vi "Save Data.vi"(0 "Which Button?":T1(ring)=enum."Center Button", 1 "start path":path, 5 "Header (If NEW is selected)":string, 7 "Data to be saved (String)":string, 9 "default name":string, 11 "error in (no error)":errorcluster) -> (4 "Maybe go back?":bool, 15 "error out":errorcluster)   [LabVIEW 2020]
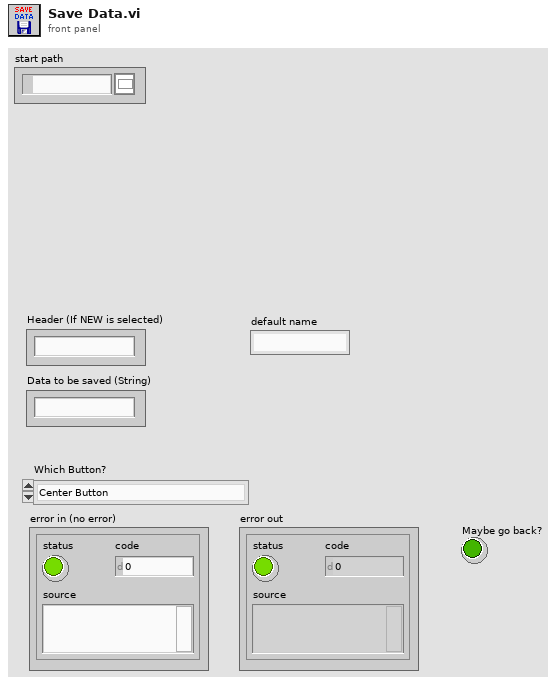
[diagram p1: front panel]
types:
  T1 = enum16{"Left Button", "Center Button", "Right Button", "Window Close"}
  T2 = enum16{"open", "replace", "create", "open or create", "replace or create", "replace or create with confirmation"}
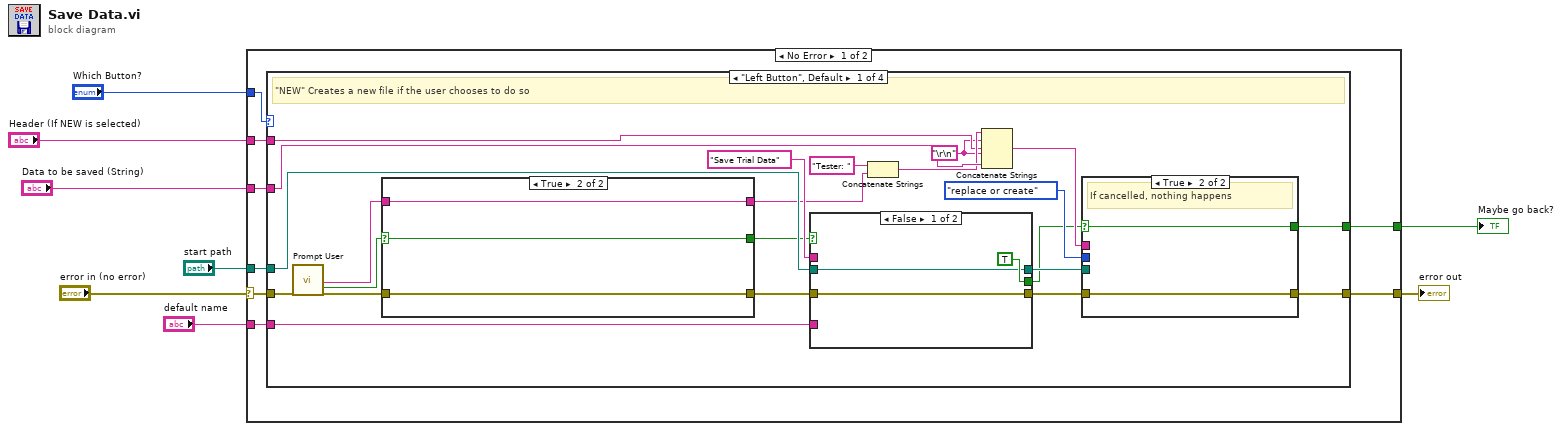
[diagram p0: block diagram]
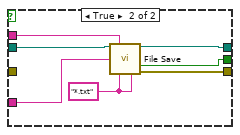
[diagram p2: hidden frame]
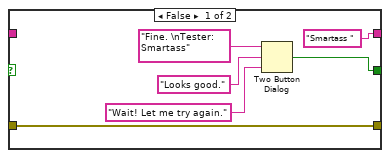
[diagram p3: hidden frame]
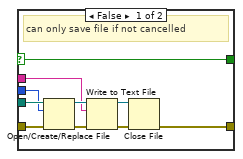
[diagram p4: hidden frame]
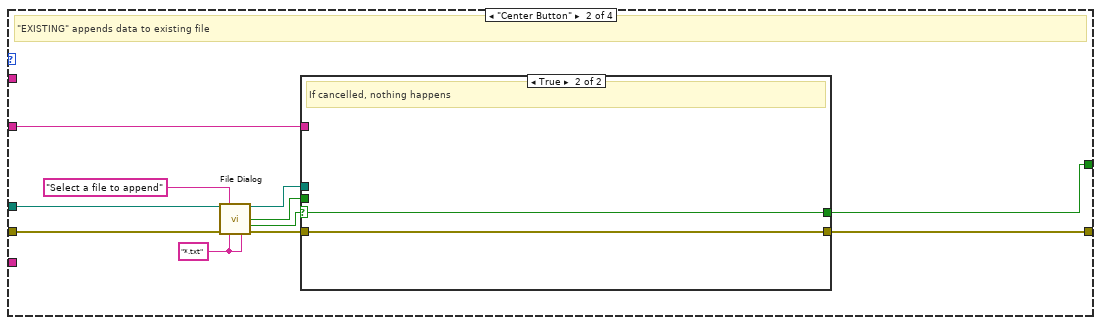
[diagram p5: hidden frame]
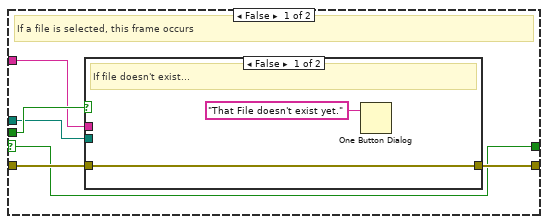
[diagram p6: hidden frame]
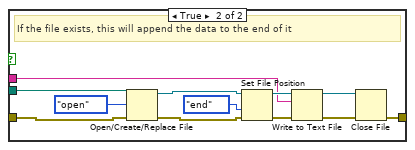
[diagram p7: hidden frame]
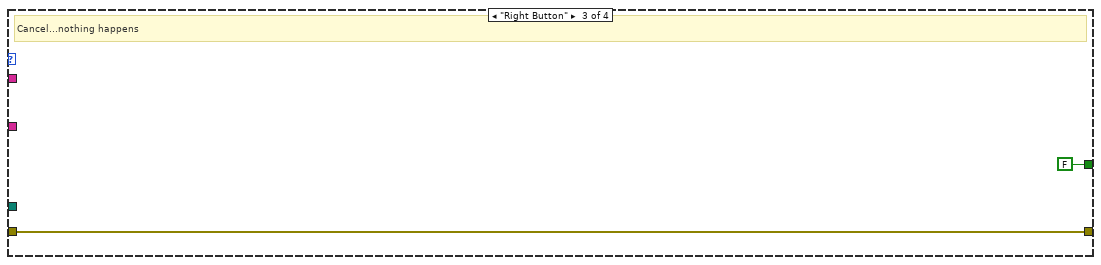
[diagram p8: hidden frame]
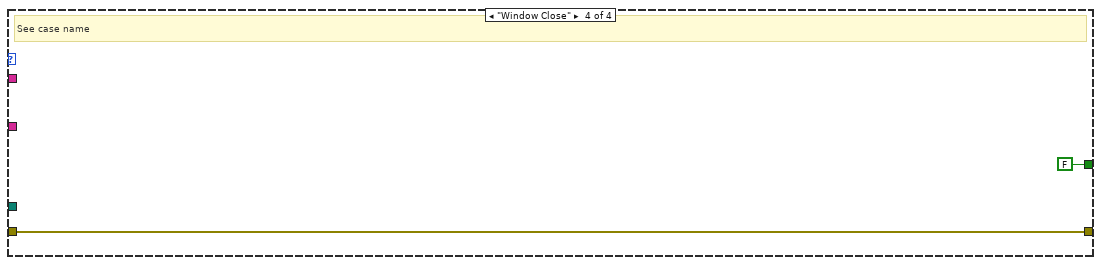
[diagram p9: hidden frame]
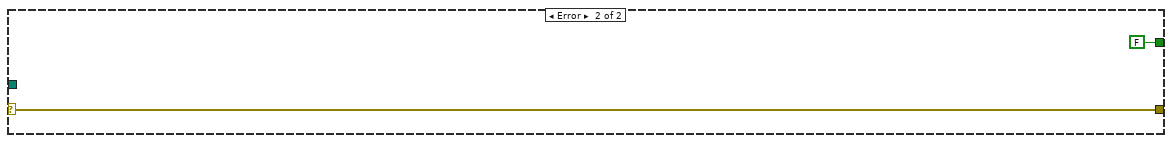
[diagram p10: hidden frame]
diagram:
  n1 = case shown="No Error" "error in (no error)" {
    selector: "error in (no error)" -> [w15 w108]
    tunnel: [w16 w108] -> w8
    tunnel: "Which Button?" -> [w14 _]
    tunnel: "Data to be saved (String)" -> [w13 _]
    tunnel: "Header (If NEW is selected)" -> [w12 _]
    tunnel: "default name" -> [w11 _]
    tunnel: [w10 FALSE] -> w2
    tunnel: "start path" -> [w9 _]
    frame No Error {
      n2 = case shown="\"Left Button\", Default" w14 {
        tunnel: w15 -> [w28 w74 w104 w106]
        tunnel: [w35 w77 w104 w106] -> w16
        tunnel: w13 -> [w33 w73 _ _]
        tunnel: w12 -> [w25 _ _ _]
        tunnel: w11 -> [w31 _ _ _]
        tunnel: [w30 w71 FALSE FALSE] -> w10
        tunnel: w9 -> [w29 w70 _ _]
        frame "Left Button", Default {
          w24 = "\r\n"
          # "\"NEW\" Creates a new file if the user chooses to do so"
          n3 = call "Prompt User"("error in (no error)"=w28) -> ("Name"=w22:string, "Done"=w23:bool, "error out"=w20:errorcluster)  [unwired: 16 in]
          n4 = case shown="True" w23 {
            selector: w23 -> [_ w56]
            tunnel: w22 -> [_ w57]
            tunnel: ["Smartass " ("string") w57] -> w21
            tunnel: [w49 w56] -> w19
            tunnel: w20 -> [w50 w55]
            tunnel: [w50 w55] -> w17
            frame False {
              n5 = Two Button Dialog(message="Fine. \nTester: Smartass", 1:"Wait! Let me try again." ("F button name (\"Cancel\")"), 2:"Looks good." ("T button name (\"OK\")")) -> (T button?=w49:bool)
            }
            frame True {
            }
          }
          n6 = case shown="False" w19 {
            tunnel: "Save Trial Data" ("prompt") -> [_ w48]
            tunnel: [w40 w47] -> w37
            tunnel: [w39 w46] -> w36
            tunnel: w31 -> [_ w45]
            tunnel: w29 -> [w39 w43]
            tunnel: [TRUE w42] -> w18
            tunnel: w17 -> [w40 _]
            frame False {
            }
            frame True {
              w44 = "*.txt" ("pattern (all files)")
              n7 = call "File Save"("start path"=w43, "prompt"=w48, "default name"=w45, "pattern (all files)"=w44, "pattern label"=w44) -> ("selected path"=w46:path, "cancelled"=w42:bool, "error out"=w47:errorcluster)  [unwired: 7 in, 1 out]
            }
          }
          n8 = Concatenate Strings("Tester: " ("string"), w21) -> (w26:string)
          n9 = Concatenate Strings(w26, w24, w25, w24, w33) -> (w32:string)
          n10 = case shown="True" w18 {
            selector: w18 -> [w58 w68]
            tunnel: w37 -> [w67 w69]
            tunnel: w36 -> [w66 _]
            tunnel: [w62 w69] -> w35
            tunnel: T2."replace or create" ("operation (0:open)") -> [w65 _]
            tunnel: w32 -> [w59 _]
            tunnel: [w58 w68] -> w30
            frame False {
              # "can only save file if not cancelled"
              n11 = Open/Create/Replace File(file path (use dialog)=w66, error in=w67, operation (0:open)=w65) -> (refnum out=w63:refnum<file>, error out=w64:errorcluster)  [unwired: 3 in, 1 out]
              n12 = Write to Text File(file (use dialog)=w63, text=w59, error in=w64) -> (refnum out=w60:refnum<file>, error out=w61:errorcluster)  [unwired: 1 in, 1 out]
              n13 = Close File(refnum=w60, error in=w61) -> (error out=w62:errorcluster)  [unwired: 1 out]
            }
            frame True {
              # "If cancelled, nothing happens"
            }
          }
        }
        frame "Center Button" {
          w72 = "*.txt" ("pattern (all files)")
          # "\"EXISTING\" appends data to existing file"
          n14 = call "File Dialog"("start path"=w70, "prompt"="Select a file to append", "error in"=w74, "pattern (all files)"=w72, "pattern label"=w72) -> ("selected path"=w75:path, "exists"=w79:bool, "cancelled"=w80:bool, "error out"=w78:errorcluster)  [unwired: 7 in]
          n15 = case shown="True" w80 {
            selector: w80 -> [w81 w101]
            tunnel: w79 -> [w86 _]
            tunnel: [w84 w102] -> w77
            tunnel: w78 -> [w85 w102]
            tunnel: w75 -> [w83 _]
            tunnel: w73 -> [w82 _]
            tunnel: [w81 w101] -> w71
            frame False {
              # "If a file is selected, this frame occurs"
              n16 = case shown="False" w86 {
                tunnel: w85 -> [w87 w100]
                tunnel: [w87 w90] -> w84
                tunnel: w83 -> [_ w98]
                tunnel: w82 -> [_ w89]
                frame False {
                  # "If file doesn't exist..."
                  n17 = One Button Dialog(message="That File doesn't exist yet.") -> ()  [unwired: 1 in, 1 out]
                }
                frame True {
                  # "If the file exists, this will append the data to the end of it"
                  n18 = Open/Create/Replace File(file path (use dialog)=w98, error in=w100, operation (0:open)=T2."open") -> (refnum out=w95:refnum<file>, error out=w97:errorcluster)  [unwired: 3 in, 1 out]
                  n19 = Set File Position(refnum=w95, from (0:start)=enum16{"start", "end", "current"}."end", error in=w97) -> (refnum out=w93:refnum<file>, error out=w94:errorcluster)  [unwired: 1 in]
                  n20 = Write to Text File(file (use dialog)=w93, text=w89, error in=w94) -> (refnum out=w91:refnum<file>, error out=w92:errorcluster)  [unwired: 1 in, 1 out]
                  n21 = Close File(refnum=w91, error in=w92) -> (error out=w90:errorcluster)  [unwired: 1 out]
                }
              }
            }
            frame True {
              # "If cancelled, nothing happens"
            }
          }
        }
        frame "Right Button" {
          # "Cancel...nothing happens"
        }
        frame "Window Close" {
          # "See case name"
        }
      }
    }
    frame Error {
    }
  }
  "error out" <- w8
  "Maybe go back?" <- w2
